vi "Acquire.vi"(6 "CurrentPad":T1, 8 "error in (no error)":errorcluster, 9 "SpectrumSat":refnum<vi>, 11 "Instruments in":refnum<class "Instruments.lvclass">) -> (0 "error out":errorcluster, 1 "20mA Spectra":cluster{"Wavelength":dbl[], "EL Spectrum":dbl[]}, 2 "Data Out":T3 {"50mA Data"."Reverse" format="%#_3g"; "50mA Data"."Current,mA" format="%_6g"; "50mA Data"."Knee Current" format="%#_3g"; "50mA Data"."WL" format="%_6g"; "50mA Data"."Voltage" format="%_6g"; "50mA Data"."Power" format="%_5g"; "20mA Data"."Reverse" format="%#_3g"; "20mA Data"."Current,mA" format="%_6g"; "20mA Data"."Knee Current" format="%#_3g"; "20mA Data"."WL" format="%_6g"; "20mA Data"."Voltage" format="%_6g"; "20mA Data"."Power" format="%_5g"}, 3 "Instruments out":refnum<class "Instruments.lvclass">, 4 "50mA Spectra":cluster{"Wavelength":dbl[], "EL Spectrum":dbl[]}, 5 "remeasure?":bool)   [LabVIEW 2012, in "Instruments.lvclass"]
uses:
  Instruments.lvclass
  Controls/TestData.ctl
  Controls/Measurement.ctl
  Controls/CurrentPad.ctl
  Controls/PadArea.ctl
  Controls/SpectrometerOphirSelector.ctl
  Instruments.lvclass/Instruments.ctl
panel:
  in  "MeasureControl":refnum<vi>
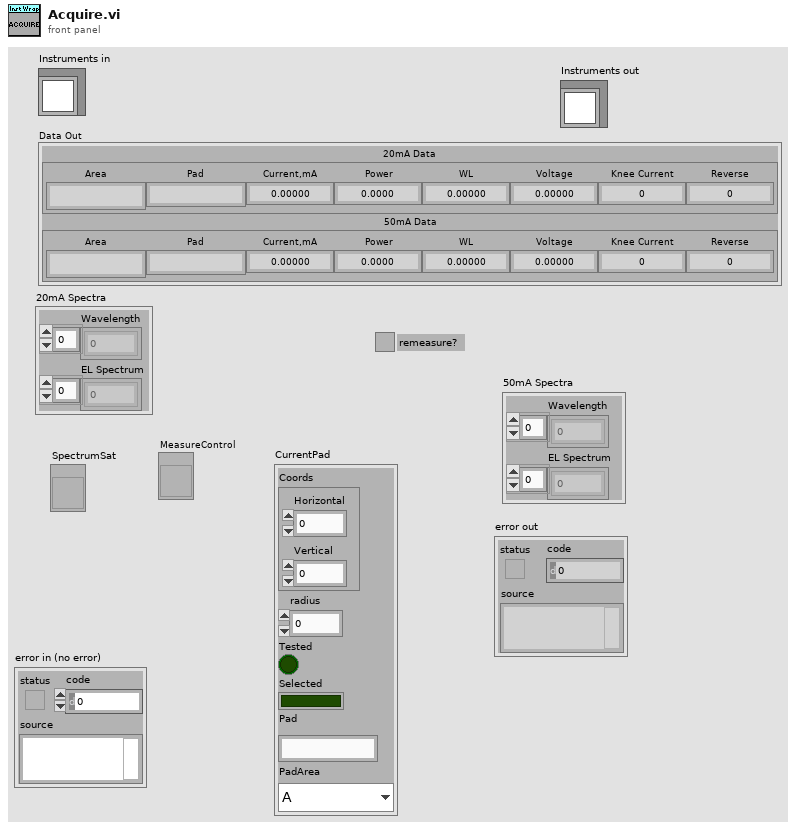
[diagram p1: front panel]
types:
  T1 = typedef "CurrentPad.ctl" = cluster{"Coords":cluster{"Horizontal":sgl, "Vertical":sgl}, "radius":i32, "Tested":bool, "Selected":bool, "Pad":string, "PadArea":T2}
  T2 = typedef "PadArea.ctl" = enum16{"A", "B", "C", "D", "L", "R", "T", "G"}
  T3 = typedef "TestData.ctl" = cluster{"20mA Data":T4, "50mA Data ":T4}
  T4 = typedef "Measurement.ctl" = cluster{"Area":string, "Pad":string, "Current,mA":dbl, "Power":dbl, "WL":dbl, "Voltage":dbl, "Knee Current":dbl, "Reverse":dbl}
  T5 = typedef "SpectrometerOphirSelector.ctl" = enum16{"Get Background", "Measure", "Measure50", "Raw"}
  T6 = typedef "MeasureControl.ctl" = cluster{"Graph":cluster{"Y":dbl[], "Y":dbl[]}[], "Pass":bool, "Fail":bool, "Measure":bool, "Wafer Area":T2, "TestData":T3, "Pad":string}
  T7 = cluster{"Wavelength":dbl[], "EL Spectrum":dbl[]}[]
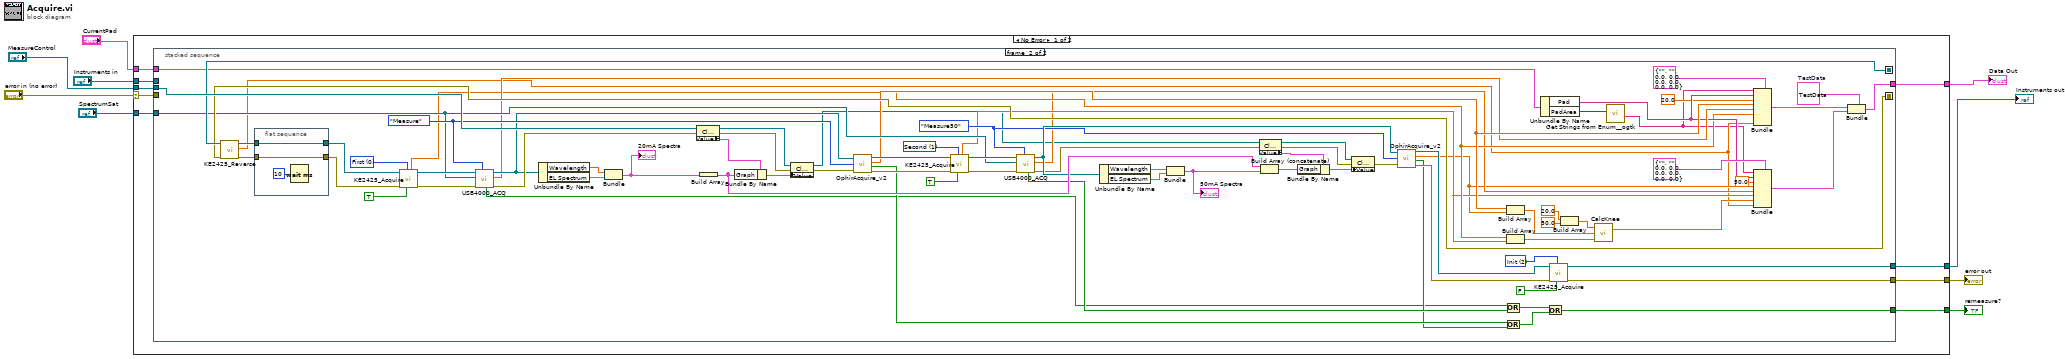
[diagram p0: block diagram]
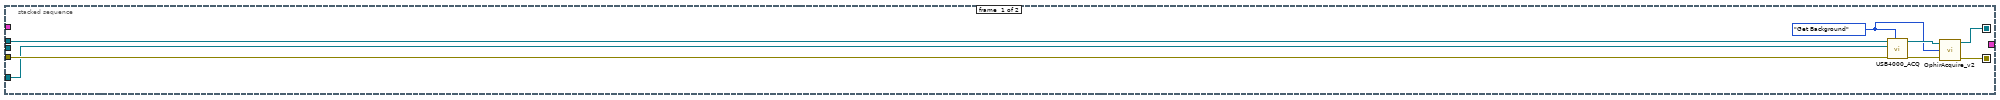
[diagram p2: hidden frame]
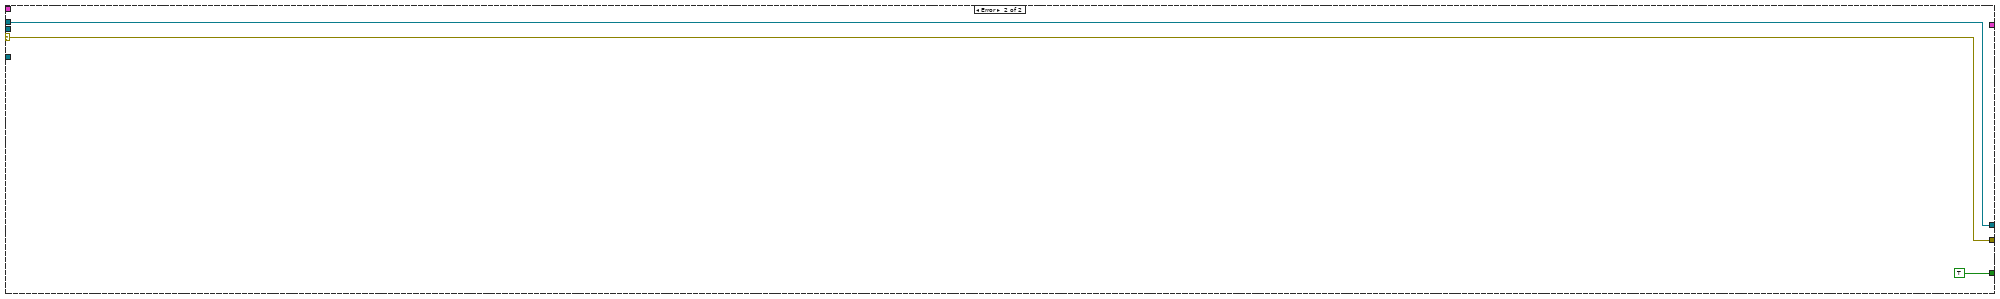
[diagram p3: hidden frame]
diagram:
  n1 = case shown="No Error" "error in (no error)" {
    selector: "error in (no error)" -> [w17 w113]
    tunnel: [w14 w113] -> w9
    tunnel: [w13 w112] -> w7
    tunnel: "Instruments in" -> [w18 w112]
    tunnel: [w16 _] -> w6
    tunnel: "MeasureControl" -> [w15 _]
    tunnel: [w12 TRUE] -> w4
    tunnel: "SpectrumSat" -> [w11 _]
    tunnel: "CurrentPad" -> [w10 _]
    frame No Error {
      n2 = stacked-sequence {
        seq-local: [w23 _] -> [_ w84]
        seq-local: [w22 _] -> [_ w83]
        tunnel: w18 -> [w26 _]
        tunnel: w17 -> [w25 _]
        tunnel: [_ w32] -> w16
        tunnel: w15 -> [_ w107]
        tunnel: [_ w71] -> w14
        tunnel: [_ w70] -> w13
        tunnel: [_ w86] -> w12
        tunnel: w11 -> [w19 w49]
        tunnel: w10 -> [_ w46]
        frame #0 {
          w20 = SpectrometerOphirSelector."Get Background" ("Type")
          n3 = call-dynamic "USB4000_ACQ.vi"("Type"=w20, "error in (no error)"=w25, "SpectrumSat"=w19, "Instruments in"=w26) -> ("error out"=w21:errorcluster, "Instruments out"=w24:refnum<class "Instruments.lvclass">)  [unwired: 4 in, 2 out]
          n4 = call-dynamic "OphirAcquire_v2.vi"("Instruments in"=w24, "Type"=w20, "error in (no error)"=w21) -> ("Instruments out"=w23:refnum<class "Instruments.lvclass">, "error out"=w22:errorcluster)  [unwired: 2 out]
        }
        frame #1 {
          w48 = T3 {"20mA Data"={"Area"="", "Pad"="", "Current,mA"=0.0, "Power"=0.0, "WL"=0.0, "Voltage"=0.0, "Knee Current"=0.0, "Reverse"=0.0}, "50mA Data "={"Area"="", "Pad"="", "Current,mA"=0.0, "Power"=0.0, "WL"=0.0, "Voltage"=0.0, "Knee Current"=0.0, "Reverse"=0.0}}  # TestData
          w58 = SpectrometerOphirSelector."Measure50" ("Type")
          w68 = SpectrometerOphirSelector."Measure" ("Type")
          w69 = u16 2 items=["First", "Second", "Init"] ("Type")
          w74 = u16 1 items=["First", "Second"] ("Type")
          w77 = u16 0 items=["First", "Second"] ("Type")
          n5 = call-dynamic "KE2425_Reverse.vi"("error in (no error)"=w83, "Instruments in"=w84) -> ("error out"=w82:errorcluster, "Current(A)"=w35:dbl, "Instruments out"=w81:refnum<class "Instruments.lvclass">)  [unwired: 6 in, 1 out]
          n6 = flat-sequence {
            tunnel: [w109] -> w80
            tunnel: w81 -> [w109]
            tunnel: w82 -> [w108]
            tunnel: [w108] -> w79
            frame #0 {
              n7 = Wait (ms)(milliseconds to wait=u32 10) -> ()  [unwired: 1 out]
            }
          }
          n8 = call-dynamic "KE2425_Acquire.vi"("KeepOn?"=TRUE ("Boolean"), "Type"=w77, "error in (no error)"=w79, "Instruments in"=w80) -> ("error out"=w78:errorcluster, "Instruments out"=w54:refnum<class "Instruments.lvclass">, "Voltage"=w41:dbl)  [unwired: 4 in, 1 out]
          n9 = call-dynamic "USB4000_ACQ.vi"("Type"=w68, "error in (no error)"=w78, "SpectrumSat"=w49, "Instruments in"=w54) -> ("error out"=w90:errorcluster, "Peak Wl"=w44:dbl, "Instruments out"=w55:refnum<class "Instruments.lvclass">, "Remeasure"=w57:bool)  [unwired: 4 in]
          n10 = Unbundle By Name(w55) -> ("Wavelength"=w53:dbl[], "EL Spectrum"=w52:dbl[])
          n11 = Bundle("Wavelength"=w53, "EL Spectrum"=w52) -> (w92:cluster{"Wavelength":dbl[], "EL Spectrum":dbl[]})  [unwired: 1 in]
          "20mA Spectra" <- w92
          n12 = property class="Clust (strict)"(reference=w107, error in=w90) -> (reference out=w104:refnum<vi>, error out=w85:errorcluster, "Value"=w106:T6)
          n13 = Build Array(w92) -> (w99:T7)
          n14 = Bundle By Name(cluster=w106, "Graph"=w99) -> (w105:T6)
          n15 = property class="Clust (strict)"(reference=w104, error in=w85, "Value"=w105) -> (reference out=w31:refnum<vi>, error out=w67:errorcluster)
          n16 = call-dynamic "OphirAcquire_v2.vi"("Instruments in"=w55, "Type"=w68, "error in (no error)"=w67) -> ("Instruments out"=w65:refnum<class "Instruments.lvclass">, "Power,uW"=w45:dbl, "Remeasure?"=w64:bool, "error out"=w66:errorcluster)
          n17 = call-dynamic "KE2425_Acquire.vi"("KeepOn?"=TRUE, "Type"=w74, "error in (no error)"=w66, "Instruments in"=w65) -> ("error out"=w75:errorcluster, "Instruments out"=w76:refnum<class "Instruments.lvclass">, "Voltage"=w38:dbl)  [unwired: 4 in, 1 out]
          n18 = call-dynamic "USB4000_ACQ.vi"("Type"=w58, "error in (no error)"=w75, "SpectrumSat"=w49, "Instruments in"=w76) -> ("error out"=w30:errorcluster, "Peak Wl"=w37:dbl, "Instruments out"=w62:refnum<class "Instruments.lvclass">, "Remeasure"=w89:bool)  [unwired: 4 in]
          n19 = Unbundle By Name(w62) -> ("Wavelength"=w51:dbl[], "EL Spectrum"=w50:dbl[])
          n20 = Bundle("Wavelength"=w51, "EL Spectrum"=w50) -> (w91:cluster{"Wavelength":dbl[], "EL Spectrum":dbl[]})  [unwired: 1 in]
          "50mA Spectra" <- w91
          n21 = property class="Clust (strict)"(reference=w31, error in=w30) -> (reference out=w102:refnum<vi>, error out=w103:errorcluster, "Value"=w100:T6)
          n22 = Build Array (concatenate)(w99, w91) -> (w98:T7)
          n23 = Bundle By Name(cluster=w100, "Graph"=w98) -> (w101:T6)
          n24 = property class="Clust (strict)"(reference=w102, error in=w103, "Value"=w101) -> (error out=w63:errorcluster)  [unwired: 1 out]
          n25 = call-dynamic "OphirAcquire_v2.vi"("Instruments in"=w62, "Type"=w58, "error in (no error)"=w63) -> ("Instruments out"=w61:refnum<class "Instruments.lvclass">, "Power,uW"=w36:dbl, "Remeasure?"=w59:bool, "error out"=w60:errorcluster)
          n26 = Or(x=w57, y=w89) -> (x .or. y?=w88:bool)
          n27 = Or(x=w64, y=w59) -> (x .or. y?=w87:bool)
          n28 = Build Array(w45, w36) -> (w94:dbl[])
          n29 = Build Array(w41, w38) -> (w93:dbl[])
          n30 = Unbundle By Name(w46) -> ("Pad"=w42:string, "PadArea"=w29:T2)
          n31 = Or(x=w88, y=w87) -> (x .or. y?=w86:bool)
          n32 = call-dynamic "KE2425_Acquire.vi"("KeepOn?"=FALSE ("source"), "Type"=w69, "error in (no error)"=w60, "Instruments in"=w61) -> ("error out"=w71:errorcluster, "Instruments out"=w70:refnum<class "Instruments.lvclass">)  [unwired: 4 in, 2 out]
          n33 = Build Array(20.0 ("input variable"), 50.0 ("input variable")) -> (w95:dbl[])
          n34 = call "CalcKnee.vi"("Voltage"=w93, "Power"=w94, "Current"=w95) -> ("Knee Current"=w39:dbl)  [unwired: 1 out]
          n35 = call <userlib>:"Get Strings from Enum__ogtk.vi"("Enum"=w29) -> ("String Value"=w28:string)  [unwired: 7 in, 3 out]
          n36 = Bundle(cluster=T4 {"Area"="", "Pad"="", "Current,mA"=0.0, "Power"=0.0, "WL"=0.0, "Voltage"=0.0, "Knee Current"=0.0, "Reverse"=0.0} ("20mA Data"), "Area"=w28, "Pad"=w42, "Current,mA"=20.0, "Power"=w45, "WL"=w44, "Voltage"=w41, "Reverse"=w35) -> (w33:T4)  [unwired: 1 in]
          n37 = Bundle(cluster=T4 {"Area"="", "Pad"="", "Current,mA"=0.0, "Power"=0.0, "WL"=0.0, "Voltage"=0.0, "Knee Current"=0.0, "Reverse"=0.0} ("20mA Data"), "Area"=w28, "Pad"=w42, "Current,mA"=50.0, "Power"=w36, "WL"=w37, "Voltage"=w38, "Knee Current"=w39, "Reverse"=w35) -> (w34:T4)
          n38 = Bundle(cluster=w48, "20mA Data"=w33, "50mA Data"=w34) -> (w32:T3)
        }
      }
    }
    frame Error {
    }
  }
  "error out" <- w9
  "Instruments out" <- w7
  "Data Out" <- w6
  "remeasure?" <- w4
